vi "Write Thermostat Target Temperature C.vi"(7 "Use Cached Data?":bool, 8 "Error In":errorcluster, 9 "Temperature (C)":dbl format="%#_13g", 10 "Device Name":string, 11 "Nest Config":T1) -> (0 "Error Out":errorcluster, 3 "Nest Config":T1)   [LabVIEW 2013, in "LVH-Nest.lvlib"]
uses:
  LVH-Nest.lvlib
  Private/Type Defs/Nest Config.ctl
  <vilib>/httpClient/ClientHandle.ctl
  Private/Type Defs/Session Data.ctl
  Private/Type Defs/Nest Error.ctl
  <vilib>/httpClient/POSTBuffer.vi
  <vilib>/httpClient/LabVIEWHTTPClient.lvlib
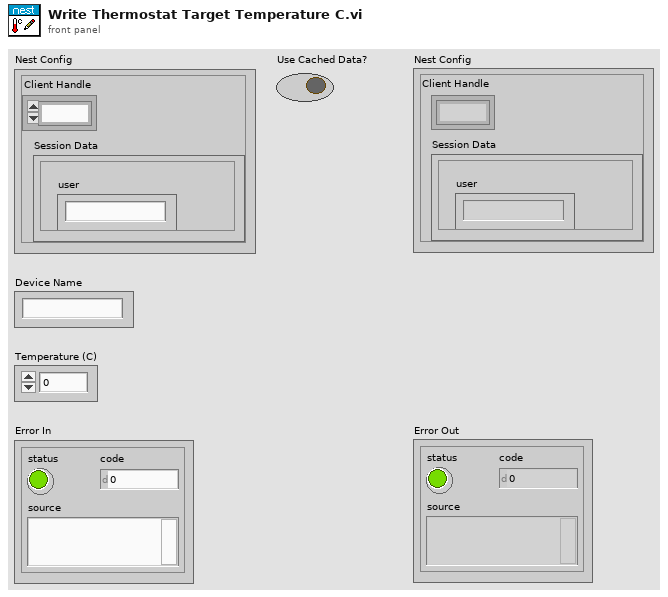
[diagram p1: front panel]
types:
  T1 = typedef "LVH-Nest.lvlib/Nest Config.ctl" = cluster{"Client Handle":T2, "Session Data":T3}
  T2 = typedef "LabVIEWHTTPClient.lvlib/ClientHandle.ctl" = refnum<k1>
  T3 = typedef "LVH-Nest.lvlib/Session Data.ctl" = cluster{"is_superuser":bool, "is_staff":bool, "urls":cluster{"transport_url":string, "rubyapi_url":string, "weather_url":string, "log_upload_url":string, "support_url":string}, "limits":cluster{"thermostats_per_structure":u32, "structures":u32, "thermostats":u32, "smoke_detectors":u32, "smoke_detectors_per_structure":u32}, "access_token":string, "userid":string, "expires_in":string, "email":string, "user":string, "language":string}
  T4 = typedef "LVH-Nest.lvlib/Nest Error.ctl" = enum16{"Unknown", "Auth", "Read", "Invalid Structure Name", "Invalid Device Name", "Set Temp"}
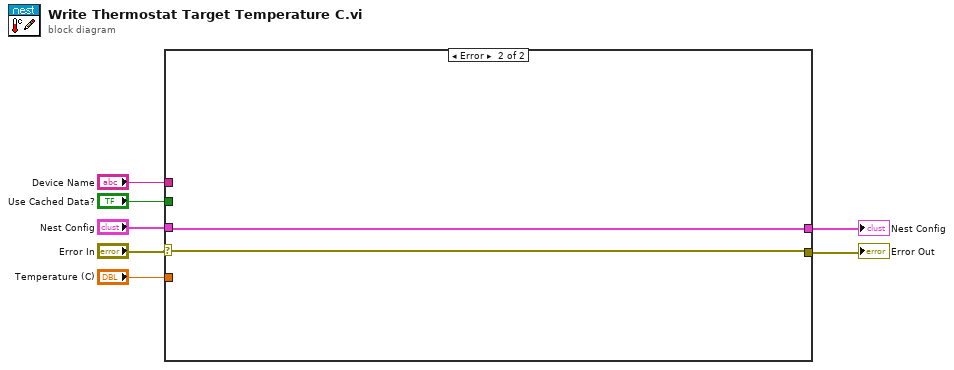
[diagram p0: block diagram]
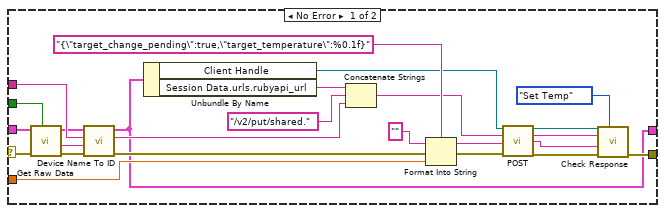
[diagram p2: hidden frame]
diagram:
  n1 = case shown="Error" "Error In" {
    selector: "Error In" -> [w30 w34]
    tunnel: "Use Cached Data?" -> [w32 _]
    tunnel: "Nest Config" -> [w31 w33]
    tunnel: "Device Name" -> [w27 _]
    tunnel: [w14 w34] -> w4
    tunnel: [w8 w33] -> w3
    tunnel: "Temperature (C)" -> [w15 _]
    frame No Error {
      n2 = call "Get Raw Data.vi"("Use Cached Data?"=w32, "Error In"=w30, "Nest Config"=w31) -> ("Error Out"=w29:errorcluster, "Data"=w28:string, "Nest Config"=w26:T1)  [unwired: 6 in]
      n3 = call "Device Name To ID.vi"("Error In"=w29, "Data"=w28, "Device Name"=w27, "Nest Config"=w26) -> ("Error Out"=w20:errorcluster, "Device ID"=w24:string, "Nest Config"=w8:T1)  [unwired: 4 in, 1 out]
      n4 = Unbundle By Name(w8) -> ("Client Handle"=w18:T2, "Session Data.urls.rubyapi_url"=w19:string)
      n5 = Concatenate Strings(w19, "/v2/put/shared.", w24) -> (w17:string)
      n6 = Format Into String(format string="{\"target_change_pending\":true,\"target_temperature\":%0.1f}", initial string="", error in=w20, w15) -> (resulting string=w16:string, error out=w22:errorcluster)
      n7 = call-poly <vilib>:"POST.vi"("client handle"=w18, "url"=w17, "buffer"=w16, "error in (no error)"=w22) -> ("client handle out"=w12:T2, "headers"=w10:string, "body"=w11:string, "error out"=w13:errorcluster)  [unwired: 8 in]
      n8 = call "Check Response.vi"("Nest Error"=Nest_Error."Set Temp", "Error In"=w13, "Body"=w11, "Header"=w10, "Client Handle"=w12) -> ("Error Out"=w14:errorcluster)  [unwired: 3 in, 3 out]
    }
    frame Error {
    }
  }
  "Error Out" <- w4
  "Nest Config" <- w3
